vi "Funktionen Schalten.vi"(8 "Fehler (Eingang)":errorcluster) -> (0 "Fehler (Ausgang)":errorcluster, 2 "Zustand":T1)   [LabVIEW 2020, in "Allgemein.lvlib"]
uses:
  Allgemein.lvlib
  Aktionen FGV Dichtheitstest.ctl
  FGV Zustaende Aktionen.ctl
  Verwaltung/Verwaltung - cRIO.lvlib
  Verwaltung/FGV OUT Aktionen.ctl
  Regler/Regler.lvlib
  Regler/FGV Daten Regler Aktionen.ctl
  Funktionstasten/Zustaende.ctl
  Funktionstasten/Funktionstasten.lvlib
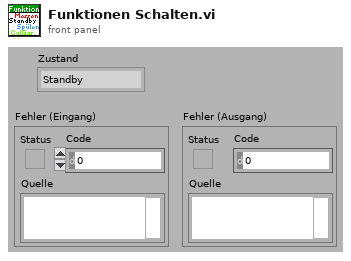
[diagram p1: front panel]
types:
  T1 = typedef "Funktionstasten.lvlib/Zustaende.ctl" = enum16{"Standby", "Pause", "Eco", "Messen", "Kalibrieren", "Spülen Filter", "Spülen Leitung", "Umgebungsluft", "0-Gas", "Cal-Gas", "CG zu PNS", "-------------", "Init 1", "Init 2", "Init 3", "Init 4", "Messen vorbereiten", "Messen durchführen", "Exit"}
  T2 = typedef "Regler.lvlib/FGV Daten Regler Aktionen.ctl" = enum16{"lesen", "Out%", "Heizung EIN"}
  T3 = typedef "Verwaltung - cRIO.lvlib/FGV OUT Aktionen.ctl" = enum16{"lesen", "ANA OUT", "DO 0-31", "DO 32-47"}
  T4 = typedef "Allgemein.lvlib/FGV Zustaende Aktionen.ctl" = enum16{"lesen", "Zustand PC", "Zustand cRIO", "Bildnummer", "Samplepoint", "Sysloglevel"}
  T5 = typedef "Allgemein.lvlib/Aktionen FGV Dichtheitstest.ctl" = enum16{"lesen", "schreiben"}
  T6 = typedef "EPA 1065.lvlib/Dichtheitstest 1065-345.lvlib/Aktion Leak check durchfuehren.ctl" = enum16{"initialisieren", "Unterdruck erzeugen", "Ventile schließen", "Warten", "Auswertung", "fertig", "PDF erstellen"}
  T7 = typedef "Erweiterte Konfig.lvlib/Aktionen Dichtheitstest.ctl" = enum16{"Initialisieren", "Unterdruck aufbauen", "Prop schließen", "Warten", "Auswertung", "Fertig"}
  T8 = cluster{"-23Y1 (CG1)":bool, "-23Y2 (CG2)":bool, "-23Y3 (CG3-10)":bool, "-23Y4 (N2)":bool, "-23Y5":bool, "-27Y2":bool, "-20Y5":bool, "-20Y6":bool, "-20Y7":bool, "-20Y8":bool, "-27Y3":bool, "-27Y4":bool, "Pumpe":bool, "Kondensat":bool, "-22Y3":bool, "-20Y2":bool, "-21Y3":bool, "Absaugung":bool, "-21Y5":bool, "CG zu Entnahme":bool, "-20Y2 (CG3)":bool, "-20Y3 (CG4)":bool, "-20Y4 (CG5)":bool, "-20Y5 (CG6)":bool, "-20Y6 (CG7)":bool, "-20Y7 (CG8)":bool, "-20Y8 (CG9)":bool, "-21Y1 (CG10)":bool}
  T9 = typedef "Verwaltung - cRIO.lvlib/Digital Ausgaenge 32-63.ctl" = cluster{"O32: Messgaspumpe EIN":bool, "O33: (Umgebungsluftpumpe)":bool, "O34: (Kondensatpumpe GK)":bool, "O35: Klima/Lüfter EIN":bool, "O36: Versorgung Heizungen":bool, "O37: Versorgung Heizungen":bool, "O38: (Gaskühler EIN (Freigabe))":bool, "O39: Störung FAS LP":bool, "O40: (Heizung Filterblock)":bool, "O41: Heizung HL zu FT-IR":bool, "O42: Heizung HL Extern SP1":bool, "O43: Heizung HL Extern SP2":bool, "O44: Heizung Reserve":bool, "O45: Heizung Reserve":bool, "O46: Statusbeleuchtung grün":bool, "O47: Statusbeleuchtung rot":bool}
  T10 = typedef "Verwaltung - cRIO.lvlib/Digital Ausgaenge 0-31.ctl" = cluster{"O0: Druckluft Versorgung":bool, "O1: CG 3 (FB Eingang 1)":bool, "O2: CG 4 (Kühlung FT-IR EIN)":bool, "O3: CG 5 (FB Bypass)":bool, "O4: CG 6 (FB CalGas)":bool, "O5: CG 7 (FB spülen/UL)":bool, "O6: CG 8 (FB zum FT-IR)":bool, "O7: CG 9 (FB zum FID)":bool, "O8: CG 10 (FB Reserve)":bool, "O9: (FB Reserve)":bool, "O10: (FB Umgebungsluft FID)":bool, "O11: (FB zum Gaskühler)":bool, "O12: FB Stickstoff zu FT-IR":bool, "O13: (FB Druckluft/UL)":bool, "O14: (Purifier deaktivieren)":bool, "O15: (Umschaltung Purifier/Stickstoff)":bool, "O16: N2 Einblasung":bool, "O17: LSP LN2 Nachfüllung":bool, "O18: (Reserve)":bool, "O19: (Pumpe Eingang1)":bool, "O20: (Pumpe Eingang2)":bool, "O21: (Pumpe Spülen1)":bool, "O22: (Pumpe Spülen2)":bool, "O23: (Reserve)":bool, "O24: CalGas 1":bool, "O25: CalGas 2":bool, "O26: CG 3-10 (CalGas 3)":bool, "O27: Stickstoff aufschalten":bool, "O28: CG zu PNS":bool, "O29: FTIR Standby Spülung":bool, "O30: CG zu Entnahme(T90)":bool, "O31: (Purifier regenerieren)":bool}
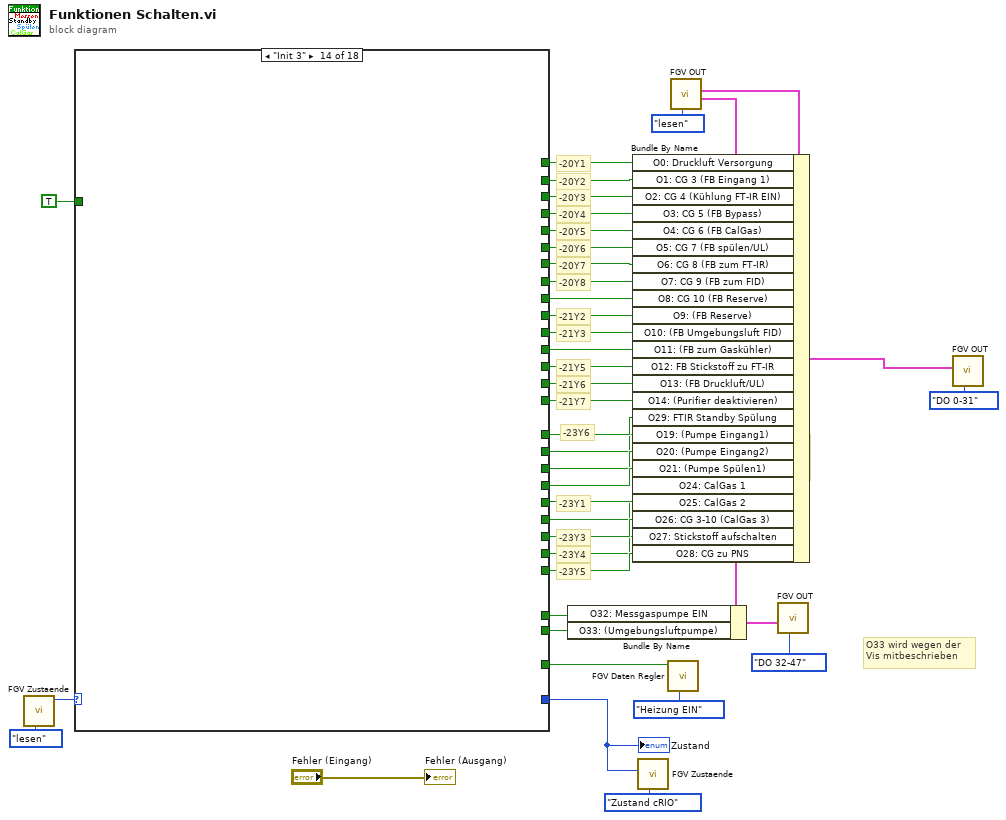
[diagram p0: block diagram]
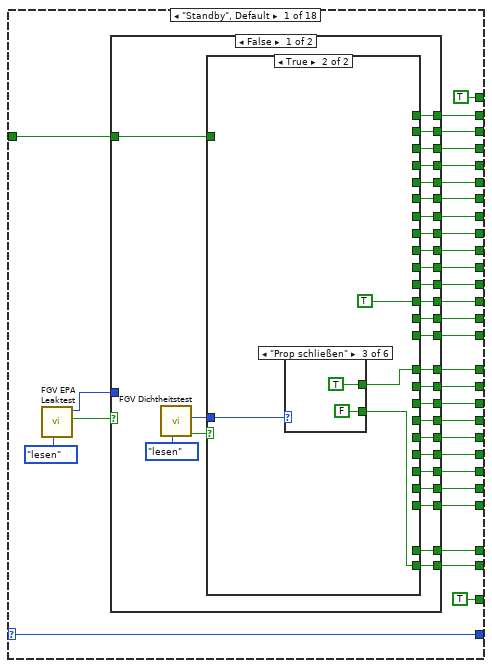
[diagram p2: hidden frame]
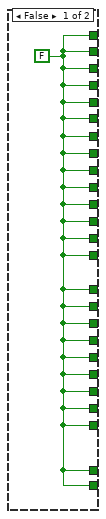
[diagram p3: hidden frame]
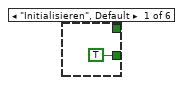
[diagram p4: hidden frame]
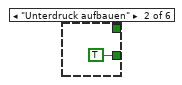
[diagram p5: hidden frame]
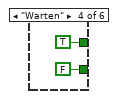
[diagram p6: hidden frame]
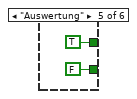
[diagram p7: hidden frame]
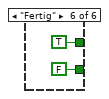
[diagram p8: hidden frame]
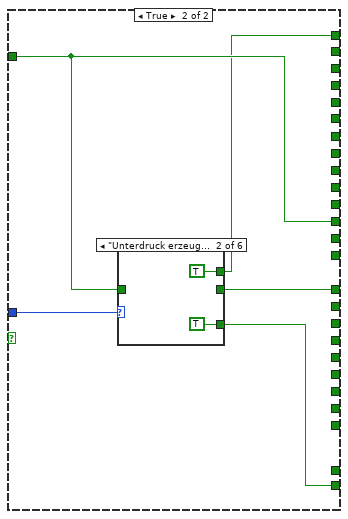
[diagram p9: hidden frame]
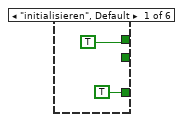
[diagram p10: hidden frame]
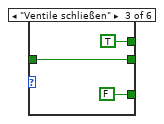
[diagram p11: hidden frame]
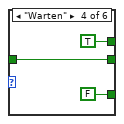
[diagram p12: hidden frame]
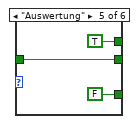
[diagram p13: hidden frame]
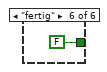
[diagram p14: hidden frame]
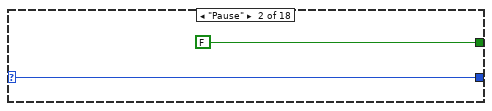
[diagram p15: hidden frame]
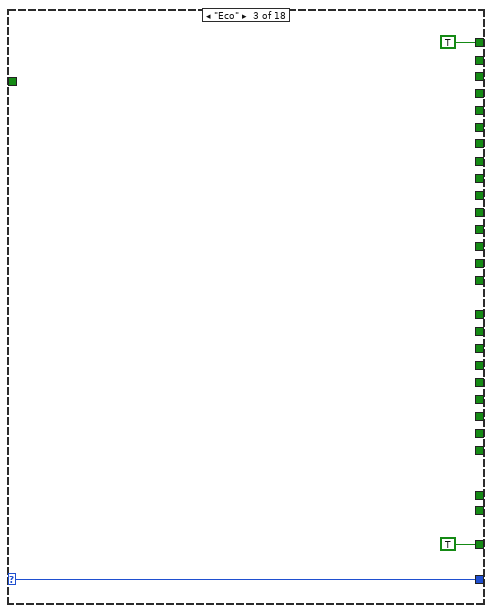
[diagram p16: hidden frame]
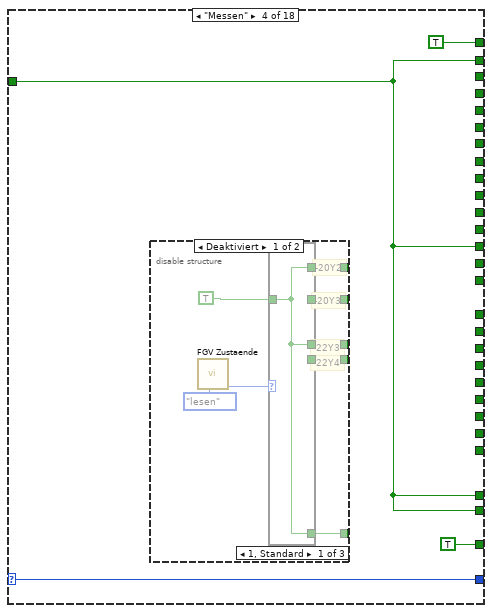
[diagram p17: hidden frame]
diagram:
  # "O33 wird wegen der \nVis mitbeschrieben"
  # "-20Y7"
  # "-23Y5"
  # "-23Y4"
  # "-20Y1"
  # "-23Y3"
  # "-22Y6"
  # "-22Y5"
  # "-22Y4"
  # "-23Y6"
  # "-21Y7"
  # "-21Y6"
  # "-21Y5"
  # "-21Y3"
  # "-21Y2"
  # "-20Y8"
  # "-20Y6"
  # "-20Y5"
  # "-20Y4"
  # "-20Y3"
  # "-20Y2"
  # "-23Y1"
  n1 = call "FGV Zustaende.vi"("Aktionen"=FGV_Zustaende_Aktionen."lesen") -> ("Zustand PC"=w16:T1)  [unwired: 6 in, 4 out]
  n2 = case shown="\"Init 3\"" w16 {
    selector: w16 -> [w73 w138 w141 w145 w167 w180 w184 w199 w216 w234 _ _ _ _ _ _ _ _]
    tunnel: [w73 w138 w141 w145 w167 w180 w184 w199 w216 w234 _ _ _ _ _ _ _ _] -> w14
    tunnel: [w71 _ _ w142 _ _ w181 _ w212 w230 _ _ _ _ _ _ _ _] -> w41
    tunnel: [w70 _ _ _ _ _ _ _ _ _ _ _ _ _ _ _ _ _] -> w40
    tunnel: [w68 _ _ _ w157 _ _ w196 w211 w229 _ _ _ _ _ _ _ _] -> w37
    tunnel: [w67 _ _ _ _ _ _ _ w210 w228 _ _ _ _ _ _ _ _] -> w36
    tunnel: [w66 _ _ _ _ _ _ _ w209 w227 _ _ _ _ _ _ _ _] -> w35
    tunnel: [w65 _ _ _ _ _ _ _ w208 w226 _ _ _ _ _ _ _ _] -> w34
    tunnel: [w64 _ _ _ _ _ _ _ _ _ _ _ _ _ _ _ _ _] -> w31
    tunnel: [w62 _ _ w142 w161 _ _ w197 w206 w225 _ _ _ _ _ _ _ _] -> w30
    tunnel: [w61 _ _ _ _ w177 w181 _ _ _ _ _ _ _ _ _ _ _] -> w27
    tunnel: TRUE -> [w72 _ _ w142 w164 w177 w181 w197 _ _ _ _ _ _ _ _ _ _]
    tunnel: [w69 _ _ _ _ w176 _ _ _ _ _ _ _ _ _ _ _ _] -> w38
    tunnel: [w60 _ _ _ _ _ _ _ _ _ _ _ _ _ _ _ _ _] -> w28
    tunnel: [w52 _ _ w142 w163 _ _ w197 w200 w220 _ _ _ _ _ _ _ _] -> w4
    tunnel: [w53 _ _ w142 _ _ _ _ _ w219 _ _ _ _ _ _ _ _] -> w5
    tunnel: [w55 _ _ _ _ _ _ _ w205 w224 _ _ _ _ _ _ _ _] -> w22
    tunnel: [w56 _ _ _ _ _ _ _ _ _ _ _ _ _ _ _ _ _] -> w25
    tunnel: [w57 _ _ _ _ _ _ _ _ _ _ _ _ _ _ _ _ _] -> w24
    tunnel: [w58 _ _ _ _ _ _ _ _ _ _ _ _ _ _ _ _ _] -> w23
    tunnel: [w59 _ _ _ w158 _ _ _ _ _ _ _ _ _ _ _ _ _] -> w26
    tunnel: [w54 _ _ _ _ _ _ _ w203 w222 _ _ _ _ _ _ _ _] -> w21
    tunnel: [TRUE ("O0: Druckluft Versorgung") _ TRUE ("O0: Druckluft Versorgung") TRUE ("O0: Druckluft Versorgung") w157 TRUE ("O0: Druckluft Versorgung") TRUE ("O0: Druckluft Versorgung") w196 TRUE ("O0: Druckluft Versorgung") TRUE ("O0: Druckluft Versorgung") _ _ _ _ _ _ _ _] -> w33
    tunnel: [w50 _ _ _ _ _ _ _ _ _ _ _ _ _ _ _ _ _] -> w32
    tunnel: [w49 _ _ _ _ _ _ _ _ _ _ _ _ _ _ _ _ _] -> w29
    tunnel: [w48 _ _ _ _ _ _ _ w204 w223 _ _ _ _ _ _ _ _] -> w20
    tunnel: [w47 _ _ _ _ _ _ _ w201 w218 _ _ _ _ _ _ _ _] -> w19
    tunnel: [w46 _ _ _ w162 _ _ w197 w202 w221 _ _ _ _ _ _ _ _] -> w18
    tunnel: [TRUE ("Heizung AUS") FALSE ("Heizung AUS") TRUE ("Heizung AUS") TRUE ("Heizung AUS") TRUE ("Heizung AUS") TRUE ("Heizung AUS") TRUE ("Heizung AUS") TRUE ("Heizung AUS") TRUE ("Heizung AUS") TRUE ("Heizung AUS") TRUE ("Heizung AUS") _ _ _ _ _ _ _] -> w6
    tunnel: [w63 _ _ _ _ _ _ _ w207 w217 _ _ _ _ _ _ _ _] -> w1
    frame "Standby", Default {
      n3 = call "FGV EPA Leaktest.vi"("Aktion"=enum16{"lesen", "schreiben"}."lesen") -> ("Leaktest aktiv"=w43:bool, "Leaktest Zustand"=w42:T6)  [unwired: 9 in]
      n4 = case shown="False" w43 {
        tunnel: w72 -> [w102 w120]
        tunnel: [w101 w119] -> w71
        tunnel: [w100 _] -> w70
        tunnel: [w99 _] -> w69
        tunnel: [w98 _] -> w68
        tunnel: [w97 _] -> w67
        tunnel: [w96 _] -> w66
        tunnel: [w95 _] -> w65
        tunnel: [w94 _] -> w64
        tunnel: [w93 _] -> w63
        tunnel: [w92 w120] -> w62
        tunnel: [w91 _] -> w61
        tunnel: [w90 _] -> w60
        tunnel: [w89 w121] -> w59
        tunnel: [w88 _] -> w58
        tunnel: [w87 _] -> w57
        tunnel: [w86 _] -> w56
        tunnel: [w85 _] -> w55
        tunnel: [w84 _] -> w54
        tunnel: [w83 _] -> w53
        tunnel: [w82 w118] -> w52
        tunnel: [w79 _] -> w50
        tunnel: [w78 _] -> w49
        tunnel: [w77 _] -> w48
        tunnel: [w76 _] -> w47
        tunnel: [w75 _] -> w46
        tunnel: w42 -> [_ w122]
        frame False {
          n5 = call "FGV Dichtheitstest.vi"("Aktionen"=Aktionen_FGV_Dichtheitstest."lesen") -> ("Dichtheitstest?"=w80:bool, "Aktionen Dichtheitstest"=w74:T7)  [unwired: 9 in]
          n6 = case shown="True" w80 {
            tunnel: [w103 _] -> w101
            tunnel: [w103 w104] -> w82
            tunnel: [w103 _] -> w83
            tunnel: [w103 _] -> w84
            tunnel: [w103 _] -> w85
            tunnel: [w103 _] -> w86
            tunnel: [w103 _] -> w87
            tunnel: [w103 _] -> w88
            tunnel: [w103 w105] -> w89
            tunnel: [w103 _] -> w90
            tunnel: [w103 _] -> w91
            tunnel: [w103 TRUE] -> w92
            tunnel: [w103 _] -> w93
            tunnel: [w103 _] -> w94
            tunnel: [w103 _] -> w95
            tunnel: [w103 _] -> w96
            tunnel: [w103 _] -> w97
            tunnel: [w103 _] -> w98
            tunnel: [w103 _] -> w99
            tunnel: [w103 _] -> w100
            tunnel: w102 -> [_ _]
            tunnel: [w103 _] -> w79
            tunnel: [w103 _] -> w78
            tunnel: [w103 _] -> w77
            tunnel: [w103 _] -> w76
            tunnel: [w103 _] -> w75
            tunnel: w74 -> [_ w106]
            frame False {
              w103 = FALSE
            }
            frame True {
              n7 = case shown="\"Prop schließen\"" w106 {
                tunnel: [_ _ TRUE TRUE TRUE TRUE] -> w105
                tunnel: [TRUE TRUE FALSE FALSE FALSE FALSE] -> w104
                frame "Initialisieren", Default {
                }
                frame "Unterdruck aufbauen" {
                }
                frame "Prop schließen" {
                }
                frame "Warten" {
                }
                frame "Auswertung" {
                }
                frame "Fertig" {
                }
              }
            }
          }
        }
        frame True {
          n8 = case shown="\"Unterdruck erzeugen\"" w122 {
            tunnel: w120 -> [_ _ w129 w132 w135 _]
            tunnel: [_ _ w129 w132 w135 _] -> w121
            tunnel: [TRUE TRUE TRUE TRUE TRUE _] -> w119
            tunnel: [TRUE TRUE FALSE FALSE FALSE FALSE] -> w118
            frame "initialisieren", Default {
            }
            frame "Unterdruck erzeugen" {
            }
            frame "Ventile schließen" {
            }
            frame "Warten" {
            }
            frame "Auswertung" {
            }
            frame "fertig" {
            }
          }
        }
      }
    }
    frame "Pause" {
    }
    frame "Eco" {
    }
    frame "Messen" {
      n9 = disable-structure shown="Deaktiviert" {
        disable-tunnel: [w153 _] -> _
        disable-tunnel: [w152 _] -> _
        disable-tunnel: [w151 _] -> _
        disable-tunnel: [w150 _] -> _
        disable-tunnel: [w149 _] -> _
        frame Disabled {
          # "-22Y4"
          # "-22Y3"
          # "-20Y2"
          # "-20Y3"
          n10 = call "FGV Zustaende.vi"("Aktionen"=FGV_Zustaende_Aktionen."lesen") -> ("Samplepoint"=w146:u16)  [unwired: 6 in, 4 out]
          n11 = case shown="1, Standard" w146 {
            tunnel: TRUE -> [w154 w155 w156]
            tunnel: [w154 _ _] -> w153
            tunnel: [w154 w155 _] -> w152
            tunnel: [_ w155 _] -> w151
            tunnel: [_ _ w156] -> w150
            tunnel: [w154 w155 _] -> w149
            frame 1, Default {
            }
            frame 2 {
            }
            frame 3 {
            }
          }
        }
        frame Enabled {
        }
      }
    }
    frame "Kalibrieren" {
      w157 = TRUE ("O0: Druckluft Versorgung")
      n12 = call "FGV Dichtheitstest.vi"("Aktionen"=Aktionen_FGV_Dichtheitstest."lesen") -> ("Dichtheitstest?"=w165:bool, "Aktionen Dichtheitstest"=w159:T7)  [unwired: 9 in]
      n13 = case shown="True" w165 {
        tunnel: w164 -> [w168 w169]
        tunnel: [w168 w169] -> w163
        tunnel: [w168 _] -> w162
        tunnel: [w168 w169] -> w161
        tunnel: w159 -> [_ w170]
        tunnel: [_ w171] -> w158
        frame False {
        }
        frame True {
          n14 = case shown="\"Initialisieren\", Standard" w170 {
            tunnel: [_ _ TRUE TRUE TRUE _] -> w171
            frame "Initialisieren", Default {
            }
            frame "Unterdruck aufbauen" {
            }
            frame "Prop schließen" {
            }
            frame "Warten" {
            }
            frame "Auswertung" {
            }
            frame "Fertig" {
            }
          }
        }
      }
    }
    frame "Spülen Filter" {
      n15 = call "Taktmerker.vi"("Aktion"=enum16{"lesen", "bearbeiten"}."lesen") -> ("1 s"=w176:bool)  [unwired: 6 in, 4 out]
    }
    frame "Spülen Leitung" {
      n16 = disable-structure shown="Deaktiviert" {
        disable-tunnel: [w192 _] -> _
        disable-tunnel: [w191 _] -> _
        disable-tunnel: [w190 _] -> _
        disable-tunnel: [w189 _] -> _
        disable-tunnel: [w188 _] -> _
        frame Disabled {
          # "-22Y6"
          # "-22Y5"
          # "-21Y7"
          # "-20Y6"
          # "-20Y3"
          n17 = call "FGV Zustaende.vi"("Aktionen"=FGV_Zustaende_Aktionen."lesen") -> ("Samplepoint"=w185:u16)  [unwired: 6 in, 4 out]
          n18 = case shown="3" w185 {
            tunnel: TRUE -> [w193 w194 w195]
            tunnel: [w193 _ _] -> w192
            tunnel: [_ w194 _] -> w191
            tunnel: [_ _ w195] -> w190
            tunnel: [_ _ w195] -> w189
            tunnel: [_ _ w195] -> w188
            frame 1, Default {
            }
            frame 2 {
            }
            frame 3 {
            }
          }
        }
        frame Enabled {
        }
      }
    }
    frame "0-Gas" {
      w196 = TRUE ("O0: Druckluft Versorgung")
    }
    frame "Cal-Gas" {
      n19 = call "CalGas aufschalten.vi"() -> ("Cluster"=w213:T8)  [unwired: 11 in]
      n20 = Unbundle By Name(w213) -> ("-20Y2"=w212:bool, "-20Y5"=w211:bool, "-20Y6"=w210:bool, "-20Y7"=w209:bool, "-20Y8"=w208:bool, "-21Y3"=w207:bool, "-21Y5"=w206:bool, "-23Y1 (CG1)"=w205:bool, "-23Y2 (CG2)"=w204:bool, "-23Y3 (CG3-10)"=w203:bool, "-23Y4 (N2)"=w202:bool, "-23Y5"=w201:bool, "Absaugung"=w200:bool)  [unwired: 5 out]
    }
    frame "CG zu PNS" {
      n21 = call "CalGas aufschalten.vi"() -> ("Cluster"=w231:T8)  [unwired: 11 in]
      n22 = Unbundle By Name(w231) -> ("-20Y2"=w230:bool, "-20Y5"=w229:bool, "-20Y6"=w228:bool, "-20Y7"=w227:bool, "-20Y8"=w226:bool, "-21Y3"=w217:bool, "-21Y5"=w225:bool, "-23Y1 (CG1)"=w224:bool, "-23Y2 (CG2)"=w223:bool, "-23Y3 (CG3-10)"=w222:bool, "-23Y4 (N2)"=w221:bool, "-23Y5"=w218:bool, "Pumpe"=w219:bool, "Absaugung"=w220:bool)  [unwired: 4 out]
    }
    frame "-------------" {
    }
    frame "Init 1" {
    }
    frame "Init 2" {
    }
    frame "Init 3" {
    }
    frame "Init 4" {
    }
    frame "Messen vorbereiten" {
    }
    frame "Messen durchführen" {
    }
    frame "Exit" {
    }
  }
  "Zustand" <- w14
  n23 = call "FGV Zustaende.vi"("Aktionen"=FGV_Zustaende_Aktionen."Zustand cRIO", "Zustand cRIO"=w14) -> ()  [unwired: 5 in, 5 out]
  n24 = call "FGV Daten Regler.vi"("Aktionen"=FGV_Daten_Regler_Aktionen."Heizung EIN", "Heizung EIN"=w6) -> ()  [unwired: 8 in, 2 out]
  n25 = call "FGV OUT.vi"("Aktion"=FGV_OUT_Aktionen."lesen") -> ("DO 32-63"=w11:T9, "DO 0-31"=w12:T10)  [unwired: 7 in, 2 out]
  n26 = Bundle By Name(cluster=w11, "O32: Messgaspumpe EIN"=w5, "O33: (Umgebungsluftpumpe)"=w4) -> (w8:T9)
  n27 = Bundle By Name(cluster=w12, "O0: Druckluft Versorgung"=w33, "O1: CG 3 (FB Eingang 1)"=w41, "O2: CG 4 (Kühlung FT-IR EIN)"=w40, "O3: CG 5 (FB Bypass)"=w38, "O4: CG 6 (FB CalGas)"=w37, "O5: CG 7 (FB spülen/UL)"=w36, "O6: CG 8 (FB zum FT-IR)"=w35, "O7: CG 9 (FB zum FID)"=w34, "O8: CG 10 (FB Reserve)"=w32, "O9: (FB Reserve)"=w31, "O10: (FB Umgebungsluft FID)"=w1, "O11: (FB zum Gaskühler)"=w29, "O12: FB Stickstoff zu FT-IR"=w30, "O13: (FB Druckluft/UL)"=w27, "O14: (Purifier deaktivieren)"=w28, "O29: FTIR Standby Spülung"=w26, "O19: (Pumpe Eingang1)"=w23, "O20: (Pumpe Eingang2)"=w24, "O21: (Pumpe Spülen1)"=w25, "O24: CalGas 1"=w22, "O25: CalGas 2"=w20, "O26: CG 3-10 (CalGas 3)"=w21, "O27: Stickstoff aufschalten"=w18, "O28: CG zu PNS"=w19) -> (w2:T10)
  n28 = call "FGV OUT.vi"("Aktion"=FGV_OUT_Aktionen."DO 32-47", "DO 32-63"=w8) -> ()  [unwired: 6 in, 4 out]
  n29 = call "FGV OUT.vi"("Aktion"=FGV_OUT_Aktionen."DO 0-31", "DO 0-31"=w2) -> ()  [unwired: 6 in, 4 out]
  "Fehler (Ausgang)" <- "Fehler (Eingang)"
